vi "servoControl.vi"() -> ()   [LabVIEW 2020]
uses:
  Global-force.vi
  Global-trigger.vi
  Global-velocity.vi
panel:
  out "pulse width (µs)":dbl
  out "global-velocity":dbl
  in  "finish":bool
  in  "return to nutral position":bool
  out "trigger":bool
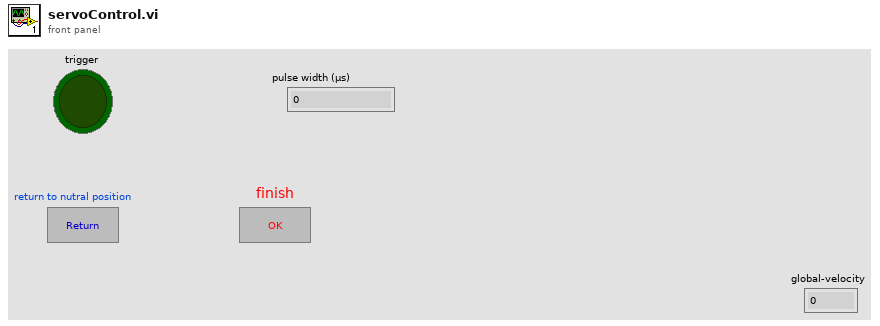
[diagram p1: front panel]
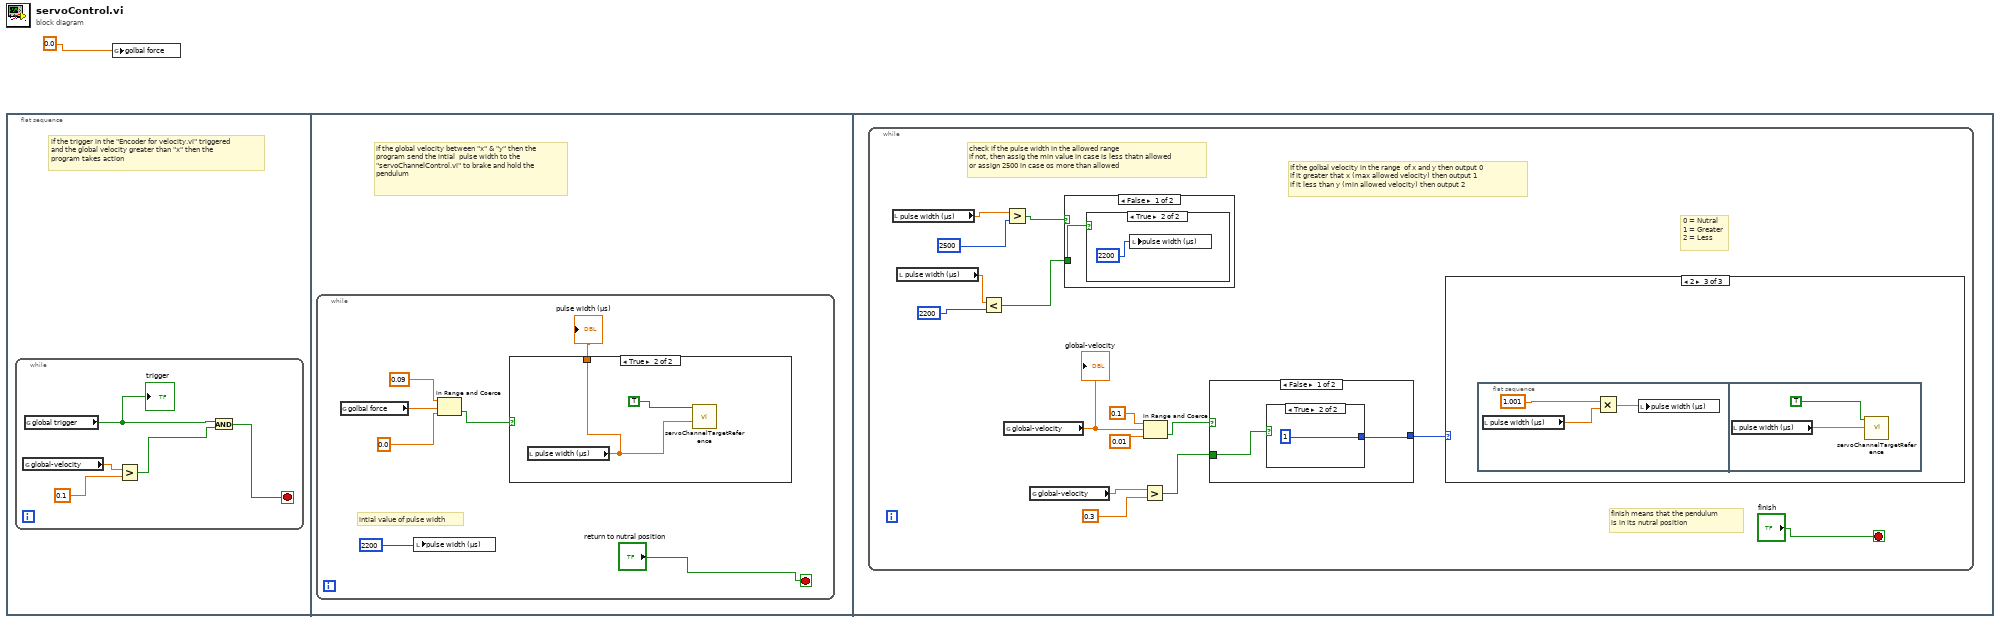
[diagram p0: block diagram]
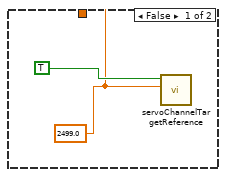
[diagram p2: hidden frame]
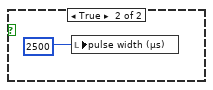
[diagram p4: hidden frame]
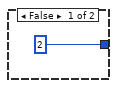
[diagram p5: hidden frame]
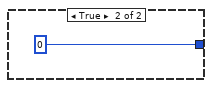
[diagram p6: hidden frame]
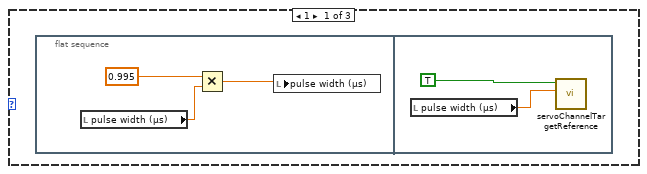
[diagram p7: hidden frame]
diagram:
  n1 = flat-sequence {
    frame #0 {
      # "if the trigger in the \"Encoder for velocity.vi\" triggered\nand the global velocity greater than \"x\" then the \nprogram takes action"
      n2 = while {
        stop <- w5 stop-if-true
        n3 = global read "Global-velocity.vi" "global-velocity"() -> (w4:dbl)
        n4 = global read "Global-trigger.vi" "global trigger"() -> (w2:bool)
        "trigger" <- w2
        n5 = Greater?(x=w4, y=0.1) -> (0:w6:bool)
        n6 = And(x=w2, y=w6) -> (x .and. y?=w5:bool)
      }
    }
    frame #1 {
      # "if the global velocity between \"x\" & \"y\" then the program send the intial  pulse width to the \"servoChannelControl.vi\" to brake and hold the pendulum"
      n7 = while {
        stop <- "return to nutral position" stop-if-true
        # "intial value of pulse width"
        n8 = global read "Global-force.vi" "golbal force"() -> (w12:dbl)
        n9 = local write "pulse width (µs)"(2200) -> ()
        n10 = In Range and Coerce(upper limit=0.09, x=w12, lower limit=0.0) -> (In Range?=w7:bool)  [unwired: 1 out]
        n11 = case shown="True" w7 {
          tunnel: [w14 w16] -> w9
          frame False {
            w14 = 2499.0
            n12 = call "servoChannelTargetReference.vi"("pulse width (µs)"=w14, "brakes on/off 2"=TRUE) -> ()  [unwired: 10 in]
          }
          frame True {
            n13 = local read "pulse width (µs)"() -> (w16:dbl)
            n14 = call "servoChannelTargetReference.vi"("pulse width (µs)"=w16, "brakes on/off 2"=TRUE) -> ()  [unwired: 10 in]
          }
        }
        "pulse width (µs)" <- w9
      }
    }
    frame #2 {
      n15 = while {
        stop <- "finish" stop-if-true
        # "check if the pulse width in the allowed range\nif not, then assig the min value in case is less thatn allowed\nor assign 2500 in case os more than allowed"
        # "0 = Nutral\n1 = Greater\n2 = Less"
        # "finish means that the pendulum \nis in its nutral position"
        # "If the golbal velocity in the range  of x and y then output 0 \nif it greater that x (max allowed velocity) then output 1\nif it less than y (min allowed velocity) then output 2"
        n16 = local read "pulse width (µs)"() -> (w23:dbl)
        n17 = local read "pulse width (µs)"() -> (w20:dbl)
        n18 = Less?(x=w20, y=2200) -> (x < y?=w18:bool)
        n19 = global read "Global-velocity.vi" "global-velocity"() -> (w29:dbl)
        "global-velocity" <- w29
        n20 = Greater?(x=w23, y=2500) -> (0:w21:bool)
        n21 = global read "Global-velocity.vi" "global-velocity"() -> (w28:dbl)
        n22 = case shown="False" w21 {
          tunnel: w18 -> [w33 _]
          frame False {
            n23 = case shown="True" w33 {
              frame False {
              }
              frame True {
                n24 = local write "pulse width (µs)"(2200) -> ()
              }
            }
          }
          frame True {
            n25 = local write "pulse width (µs)"(2500) -> ()
          }
        }
        n26 = Greater?(x=w28, y=0.3) -> (0:w24:bool)
        n27 = In Range and Coerce(upper limit=0.1, x=w29, lower limit=0.01) -> (In Range?=w26:bool)  [unwired: 1 out]
        n28 = case shown="False" w26 {
          tunnel: [w36 i8 0] -> w25
          tunnel: w24 -> [w37 _]
          frame False {
            n29 = case shown="True" w37 {
              tunnel: [i8 2 i8 1] -> w36
              frame False {
              }
              frame True {
              }
            }
          }
          frame True {
          }
        }
        n30 = case shown="2" w25 {
          frame 1 {
            n31 = flat-sequence {
              frame #0 {
                n32 = local read "pulse width (µs)"() -> (w41:dbl)
                n33 = Multiply(x=0.995, y=w41) -> (x*y=w42:dbl)
                n34 = local write "pulse width (µs)"(w42) -> ()
              }
              frame #1 {
                n35 = local read "pulse width (µs)"() -> (w45:dbl)
                n36 = call "servoChannelTargetReference.vi"("pulse width (µs)"=w45, "brakes on/off 2"=TRUE ("brakes on/off")) -> ()  [unwired: 10 in]
              }
            }
          }
          frame 0, Default {
            # "do nothing"
          }
          frame 2 {
            n37 = flat-sequence {
              frame #0 {
                n38 = local read "pulse width (µs)"() -> (w48:dbl)
                n39 = Multiply(x=1.001, y=w48) -> (x*y=w46:dbl)
                n40 = local write "pulse width (µs)"(w46) -> ()
              }
              frame #1 {
                n41 = local read "pulse width (µs)"() -> (w50:dbl)
                n42 = call "servoChannelTargetReference.vi"("pulse width (µs)"=w50, "brakes on/off 2"=TRUE) -> ()  [unwired: 10 in]
              }
            }
          }
        }
      }
    }
  }
  n43 = global write "Global-force.vi" "golbal force"(0.0) -> ()
